vi "Read Power Setpoint (Single).vi"(8 "error in":errorcluster, 10 "Channel Index":i32=1, 11 "Power Control in":refnum<class "Power Control.lvclass">) -> (0 "error out":errorcluster, 1 "Changed or First Call?":bool, 2 "Power Setpoint":dbl, 3 "Power Control out":refnum<class "Power Control.lvclass">)   [LabVIEW 2023, in "Power Control.lvclass"]
doc: "This VI will read a single Channel's setpoint. The <b>Channel Index</b> input is 1-based."
uses:
  Power Control.lvclass
  Power Control.lvclass/Power Control.ctl
  <vilib>/ADAS Replay HIL/Channels/Tag Wrapper/Polymorphic/Read Channel (Double).vi
  af94bebd-7708-4158-8814-30f53347f523.vi
  <vilib>/ADAS Replay HIL/Channels/Tag Wrapper/Polymorphic/Read Channel (Double).vi/b2f764de-0c1e-4784-a155-687fc995a684.vi
  <vilib>/ADAS Replay HIL/Channels/Tag Wrapper/Polymorphic/Read Channel (Double).vi/b2f764de-0c1e-4784-a155-687fc995a684.vi/c28b0ead-42ad-4072-80a2-aca7f2bd7ce3.vi
  <vilib>/ADAS Replay HIL/Channels/Tag Wrapper/Polymorphic/Read Channel (Double).vi/b2f764de-0c1e-4784-a155-687fc995a684.vi/219d0231-d98b-4193-b5cc-84f90e3c9091.vi
  <vilib>/ADAS Replay HIL/Channels/Tag Wrapper/Tag Wrapper.lvlib
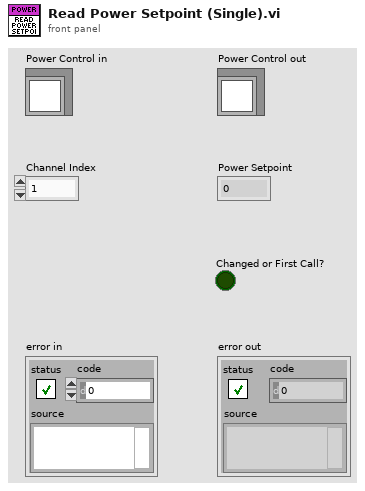
[diagram p1: front panel]
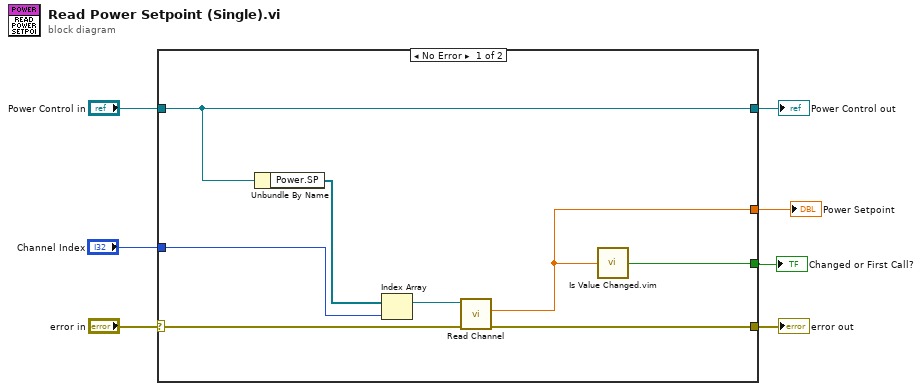
[diagram p0: block diagram]
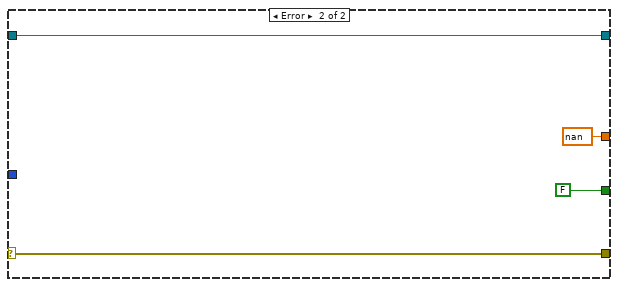
[diagram p2: hidden frame]
diagram:
  n1 = case shown="No Error" "error in" {
    selector: "error in" -> [w15 w19]
    tunnel: [w13 w19] -> w6
    tunnel: [w14 w18] -> w4
    tunnel: "Power Control in" -> [w14 w18]
    tunnel: [w11 nan ("Value out")] -> w3
    tunnel: [w10 FALSE ("changed or first call?")] -> w2
    tunnel: "Channel Index" -> [w8 _]
    frame No Error {
      n2 = Unbundle By Name(w14) -> ("Power.SP"=w12:refnum<k21>[])
      n3 = Index Array(array=w12, index=w8) -> (element=w9:refnum<k21>)
      n4 = call-poly <vilib>:"Read Channel.vi"("error in"=w15, "ADAS HIL Channel in"=w9) -> ("error out"=w13:errorcluster, "Value out"=w11:dbl)  [unwired: 6 in, 2 out]
      n5 = call "Is Value Changed.vim"("value"=w11) -> ("changed or first call?"=w10:bool)
    }
    frame Error {
    }
  }
  "error out" <- w6
  "Power Control out" <- w4
  "Power Setpoint" <- w3
  "Changed or First Call?" <- w2
